vi "Mode 1 & 2.vi"() -> ()   [LabVIEW 2020]
uses:
  <vilib>/Platform/TimedLoop/XDataNode/timing_clust.ctl
  <vilib>/Platform/TimedLoop/XDataNode/nitl_modes.ctl
  <vilib>/Platform/TimedLoop/XDataNode/wakeup.ctl
  <vilib>/MakerHub/LINX/Public/Peripherals/Digital/Digital Read N Chans.vi
  <vilib>/MakerHub/LINX/Public/Peripherals/PWM/PWM Set Duty Cycle 1 Chan.vi
  <vilib>/MakerHub/LINX/Public/Peripherals/Digital/Digital Write N Chans.vi
  <vilib>/MakerHub/LINX/Private/Local IO/LinxDigitalRead.vi
  <vilib>/MakerHub/LINX/Public/Utilities/Check Channel.vi
  <vilib>/MakerHub/LINX/Private/Local IO/LinxDigitalWrite.vi
  <vilib>/MakerHub/LINX/Public/Utilities/Open Serial.vi
  <vilib>/MakerHub/LINX/Private/Utilties/Generate Error.vi
  <vilib>/MakerHub/LINX/Public/Peripherals/PWM/PWM Set Duty Cycle N Chans.vi
  <vilib>/MakerHub/LINX/Public/Sensors/Motion/Servo/Servo Open N Channels.vi
  <vilib>/MakerHub/LINX/Public/Sensors/Motion/Servo/Servo Set Pulse Width One Channel.vi
  <vilib>/MakerHub/LINX/Public/Sensors/Motion/Servo/Servo Close N Channels.vi
  <vilib>/platform/TimedLoop/XDataNode/XDataNode.xnode
  <vilib>/MakerHub/LINX/LMH-LINX.lvlib
  <vilib>/Platform/TimedLoop/XDataNode/XDNodeRunTimeDep.lvlib
  <vilib>/MakerHub/LINX/Public/Sensors/Motion/Servo/Servo.lvlib
panel:
  in  "Titik Stop":u16=110
  in  "Point":i32
  in  "Start Main Program":bool
  in  "Servo Magazine Pin":u8=3
  in  "Servo Slider 2 Pin":u8=4
  in  "Servo Slider 1 Pin":u8=5
  in  "Values":bool[](array[boolean])
  in  "Servo Slider 2 Angle":u16(knob)=82 scale=0.0..180.0
  in  "Servo Slider 1 Angle":u16(knob)=84 scale=0.0..180.0
  in  "Servo Magazine Angle":u16(knob)=110 scale=0.0..180.0
  in  "Slider Counter":dbl[](array[numeric])=[0.0, 0.0, 0.0, 13.0]
  out "Non-metal Workpiece":bool
  out "Metal Workpiece":bool
  out "Black Workpiece":bool
  out "White Workpiece":bool
  in  "Main Program":T1(array[cluster])=[{"Mode"=enum."Idle", "Limit"=enum."Tidak Ada", "Delay"=0, "Point"=0, "Row"=0}, {"Mode"=enum."Cek Ketersediaan", "Limit"=enum."Tidak Ada", "Delay"=500, "Point"=0, "Row"=1}, {"Mode"=enum."Workpiece Masuk", "Limit"=enum."Tidak Ada", "Delay"=0, "Point"=0, "Row"=2}, {"Mode"=enum."Cek Warna", "Limit"=enum."Tidak Ada", "Delay"=1000, "Point"=0, "Row"=3}, {"Mode"=enum."Cek Counter", "Limit"=enum."Tidak Ada", "Delay"=1000, "Point"=0, "Row"=4}, {"Mode"=enum."Servo Set", "Limit"=enum."Tidak Ada", "Delay"=1000, "Point"=0, "Row"=5}, {"Mode"=enum."Conveyor Jalan", "Limit"=enum."Tidak Ada", "Delay"=0, "Point"=0, "Row"=6}, {"Mode"=enum."Servo Reset", "Limit"=enum."Tidak Ada", "Delay"=1000, "Point"=0, "Row"=7}, {"Mode"=enum."Counter", "Limit"=enum."Tidak Ada", "Delay"=0, "Point"=0, "Row"=8}, {"Mode"=enum."Go To", "Limit"=enum."Tidak Ada", "Delay"=0, "Point"=1, "Row"=9}, {"Mode"=enum."Idle", "Limit"=enum."Tidak Ada", "Delay"=0, "Point"=0, "Row"=0}, {"Mode"=enum."Idle", "Limit"=enum."Tidak Ada", "Delay"=0, "Point"=0, "Row"=0}, {"Mode"=enum."Idle", "Limit"=enum."Tidak Ada", "Delay"=0, "Point"=0, "Row"=0}]
  in  "Stop Main Program":bool
  out "Row":i32
  in  "STOP":bool
  in  "Speed Pin":u8=2
  in  "Sensor Pin":u8[](array[numeric])=[30, 32, 50, 34, 36, 38]
  out "Sensor Value":bool[](array[boolean])
  in  "Duty Cycle":dbl(knob) scale=0.0..100.0
  out "Device Name":string
  in  "Arduino Port":refnum<visa-resource-name>="N/A"
  # "LOW COST MPS SORTING BASED ARDUINO"
  # "MAIN PROGRAM"
  # "PROJECT MONITOR"
  # "MODE 1"
  # "Index Array Counter\n\n-----Mode 1-----\n0. White Workpiece          \n1. Black Workpiece\n\n-----Mode 2-----\n0. Metal Workpiece\n1. Non-metal Workpiece"
  # "MODE 2"
  # "INPUT/OUTPUT CONTROL"
  # "Index Array Input Sensor\n\n0. IR Sensor Stack Magazine\n1. IR Sensor B/W Check\n2. Inductive Proximity Sensor\n3. IR Sensor Slider 1\n4. IR Sensor Slider 2\n5. IR Sensor Slider 3"
  # "Mechatronics Engineering 2nd Generation - Vocational High School 2 Bojonegoro"
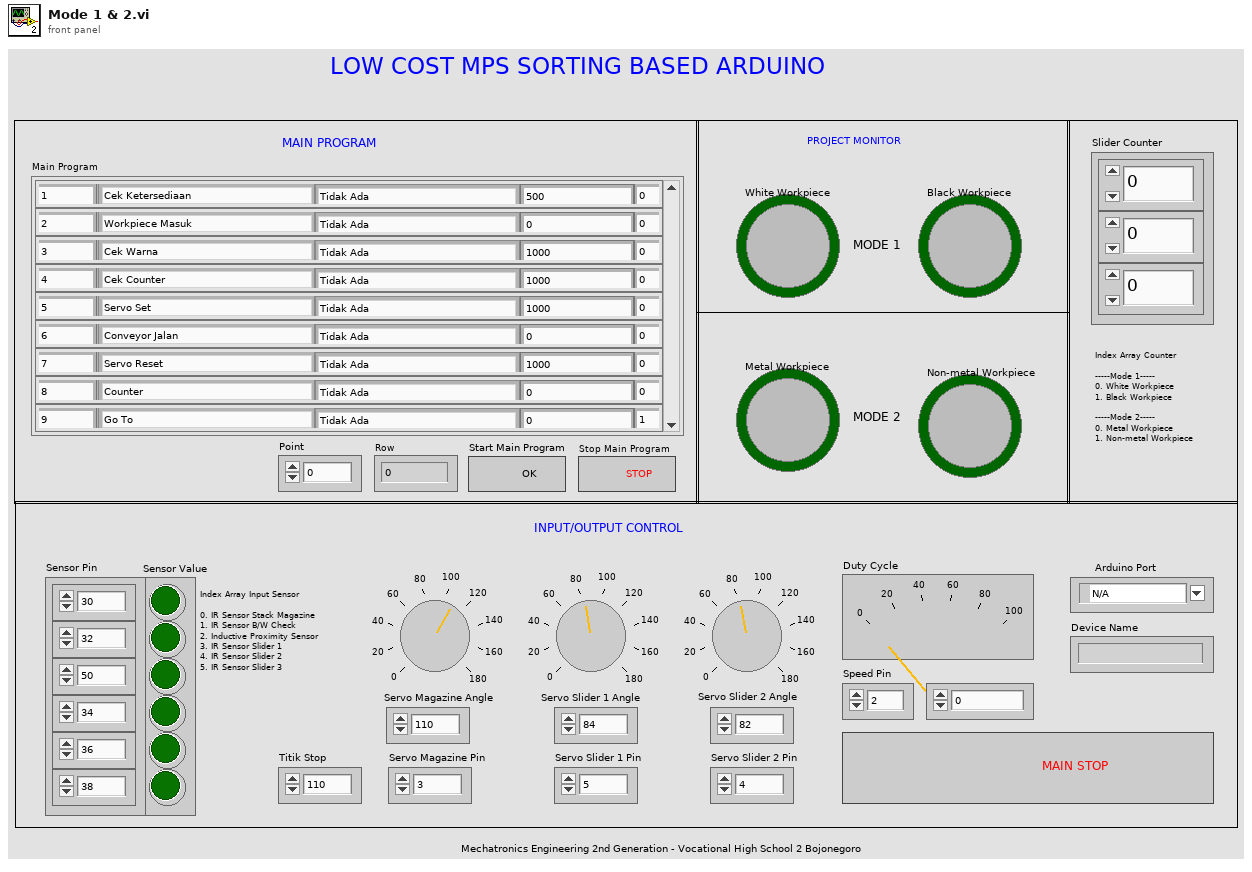
[diagram p1: front panel]
types:
  T1 = cluster{"Mode":enum16{"Idle", "Cek Ketersediaan", "Workpiece Masuk", "Cek Bahan", "Cek Warna", "Servo Set", "Conveyor Jalan", "Servo Reset", "Counter", "Cek Counter", "Go To"}, "Limit":enum16{"Tidak Ada", "Sensor Slider"}, "Delay":i32, "Point":i32, "Row":i32}[]
  T2 = typedef "XDNodeRunTimeDep.lvlib/timing_clust.ctl" = cluster{"Expected End [f-1]":u64, "Actual End [f-1]":u64, "Finished Late? [f-1]":bool, "Expected End [i-1]":u64, "Actual End [i-1]":u64, "Finished Late? [i-1]":bool, "Expected Start [i]":u64, "Actual Start [i]":u64, "Expected Start [f]":u64, "Actual Start [f]":u64, "Source Name":string, "Structure Name":string, "Period":i64, "Deadline":i64, "Offset":i64, "Start":i64, "Priority":i32, "Timeout":i32, "Mode":T3, "Wakeup Reason":T4, "Error":errorcluster, "Source Type":string, "Secondary Source Type":string, "Global End Time":u64, "Global Start Time":u64, "Frame Duration":u64, "Iteration Duration":u64, "Assigned CPU":i32, "I/O Scan Engine Mode":u32}
  T3 = typedef "XDNodeRunTimeDep.lvlib/nitl_modes.ctl" = enum32{"No Change", "Process missed periods, maintain original phase", "Discard missed periods, maintain original phase", "Process missed periods, ignore original phase", "Discard missed periods, ignore original phase"}
  T4 = typedef "XDNodeRunTimeDep.lvlib/wakeup.ctl" = enum32{"Normal", "Aborted", "Asynchronous wakeup", "Timing source error", "Timed loop error", "Timeout"}
  T5 = cluster{"Mode":enum16{"Idle", "Cek Ketersediaan", "Workpiece Masuk", "Cek Bahan", "Cek Warna", "Servo Set", "Conveyor Jalan", "Servo Reset", "Counter", "Cek Counter", "Go To"}, "Limit":enum16{"Tidak Ada", "Sensor Slider"}, "Delay":i32, "Point":i32, "Row":i32}
  T6 = enum16{"Idle", "Cek Ketersediaan", "Workpiece Masuk", "Cek Bahan", "Cek Warna", "Servo Set", "Conveyor Jalan", "Servo Reset", "Counter", "Cek Counter", "Go To"}
  T7 = typedef "LMH-LINX.lvlib/LINX Ref.ctl" = cluster{"IO":T8, "Interface":T9, "LINX Device Config":T10}
  T8 = typedef "LMH-LINX.lvlib/Platform.ctl" = enum16{"Remote", "Local"}
  T9 = typedef "LMH-LINX.lvlib/Interface.ctl" = enum16{"Serial", "TCP"}
  T10 = typedef "LMH-LINX.lvlib/Device.lvlib/LINX Device Config.ctl" = cluster{"Interface":T9, "COM Port":refnum<visa-resource-name>, "TCP Configuration":T11, "Device Family":u8, "Device ID":u8, "Device Name":string, "TCP Ref":refnum<k5>, "Channels":T12}
  T11 = typedef "LMH-LINX.lvlib/Device.lvlib/TCP Config.ctl" = cluster{"IP Address":string, "Port":u16}
  T12 = typedef "LMH-LINX.lvlib/Channels.ctl" = cluster{"DI":u8[], "DO":u8[], "AI":u8[], "AO":u8[], "PWM":u8[], "QE":u8[], "UART":u8[], "I2C 2":u8[], "SPI":u8[], "CAN":u8[], "Servo":u8[], "AI Ref (V)":dbl, "AI Resolution (Bits)":u8, "AO Ref (V)":dbl, "AO Resolution (Bits)":u8}
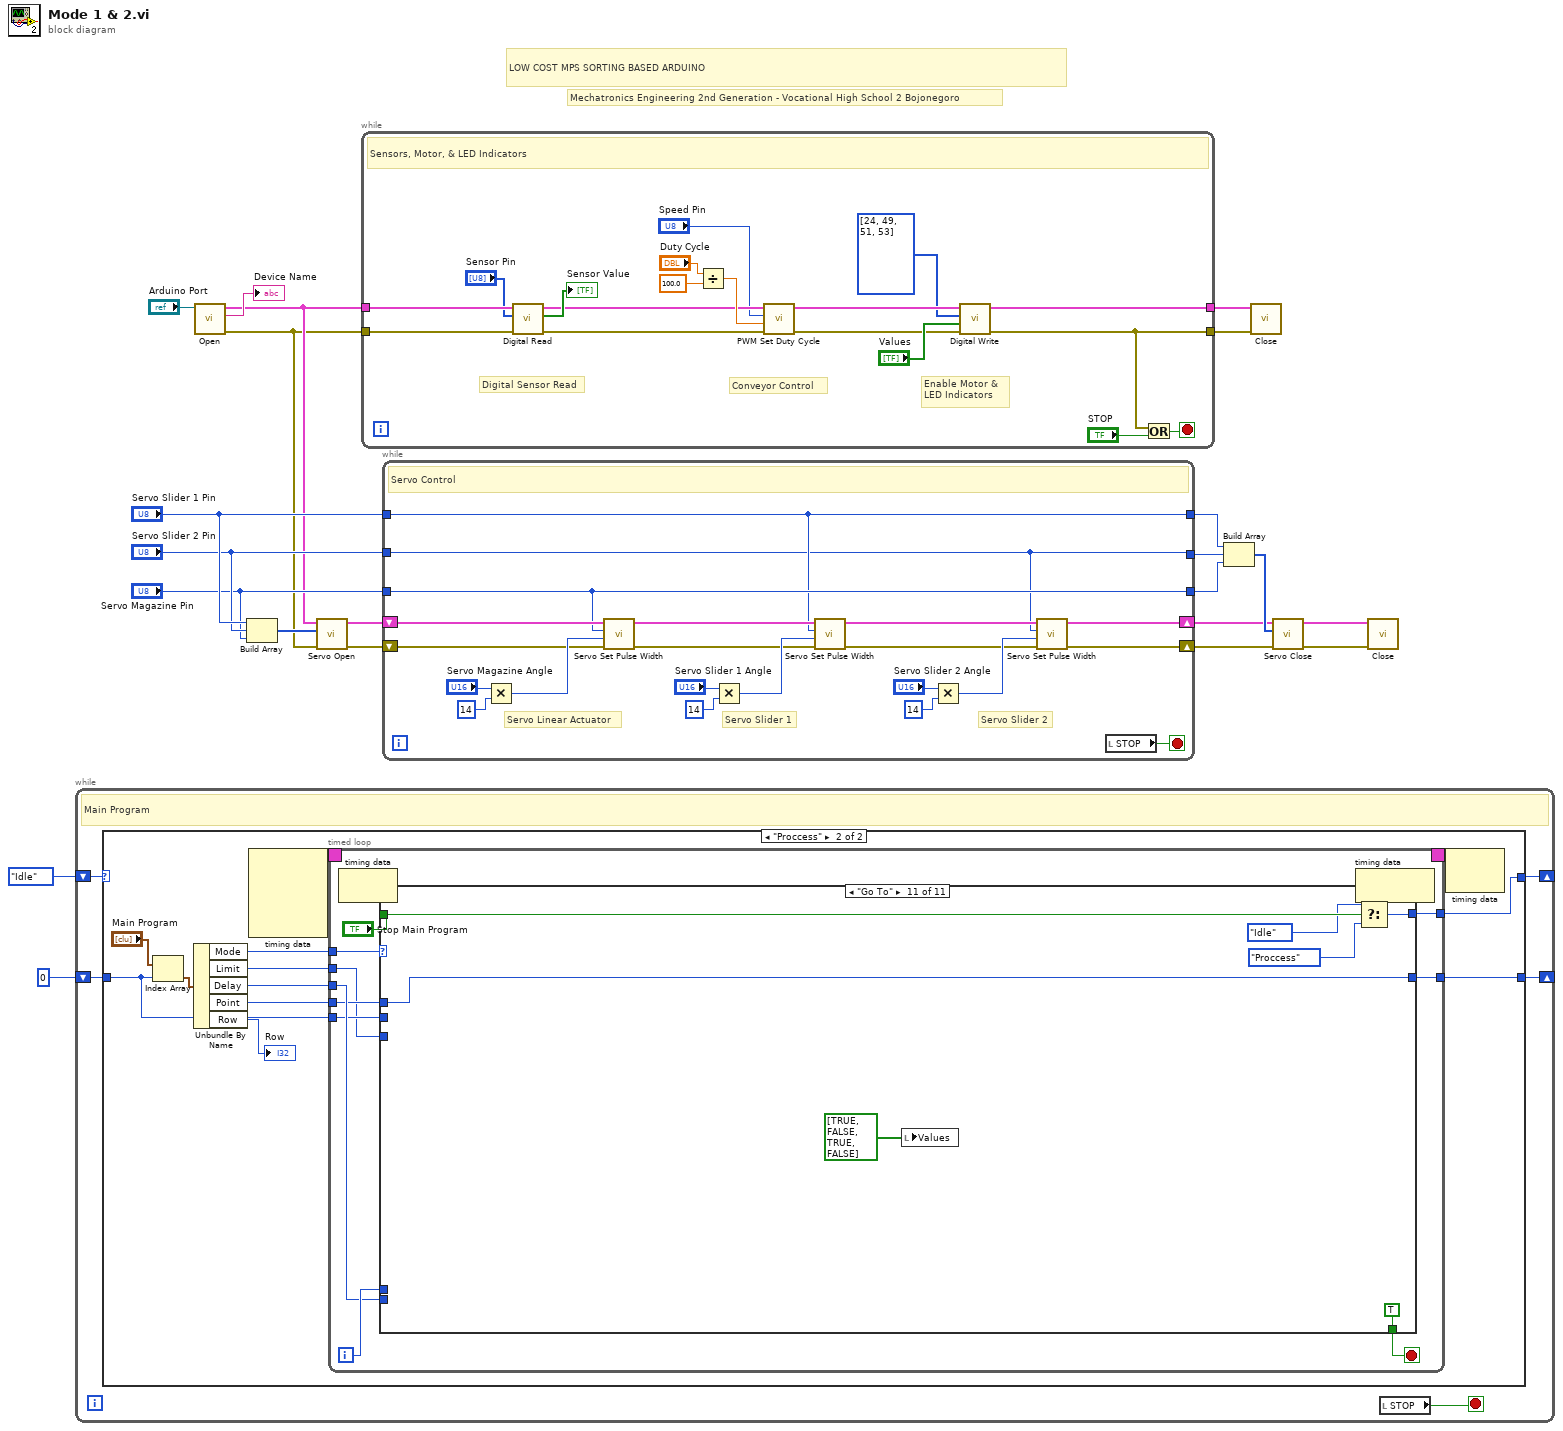
[diagram p0: block diagram]
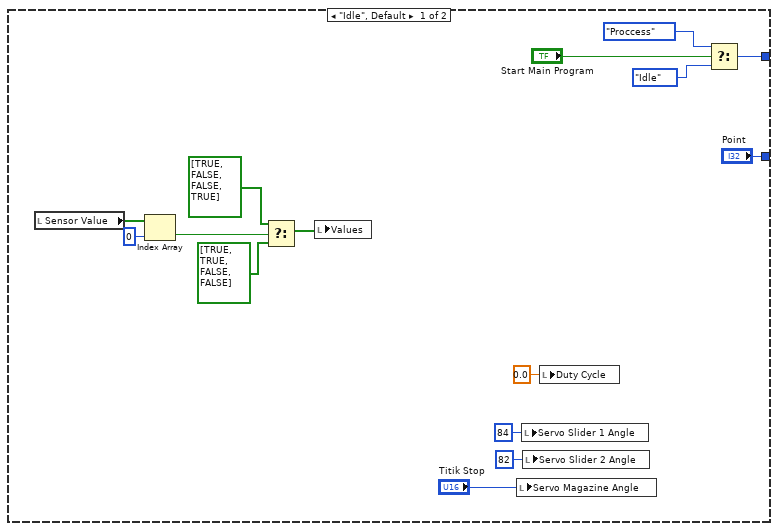
[diagram p2: hidden frame]
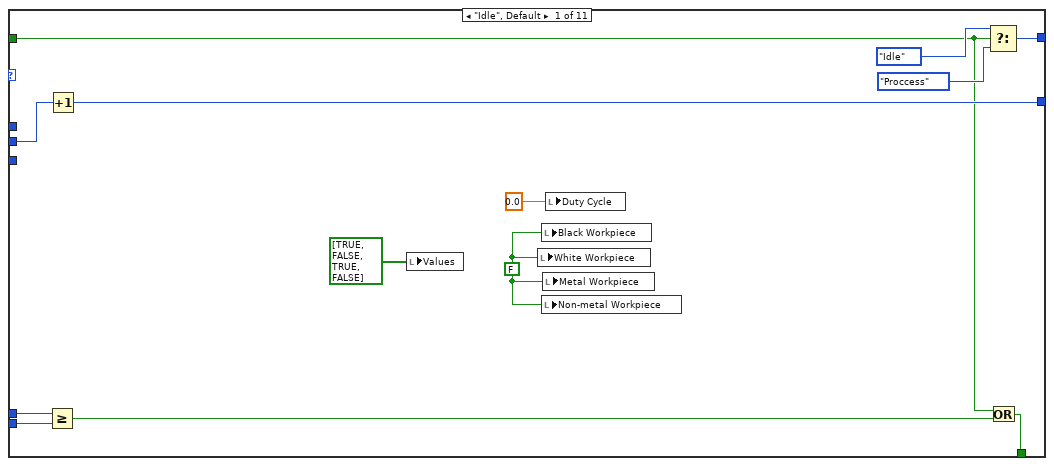
[diagram p3: hidden frame]
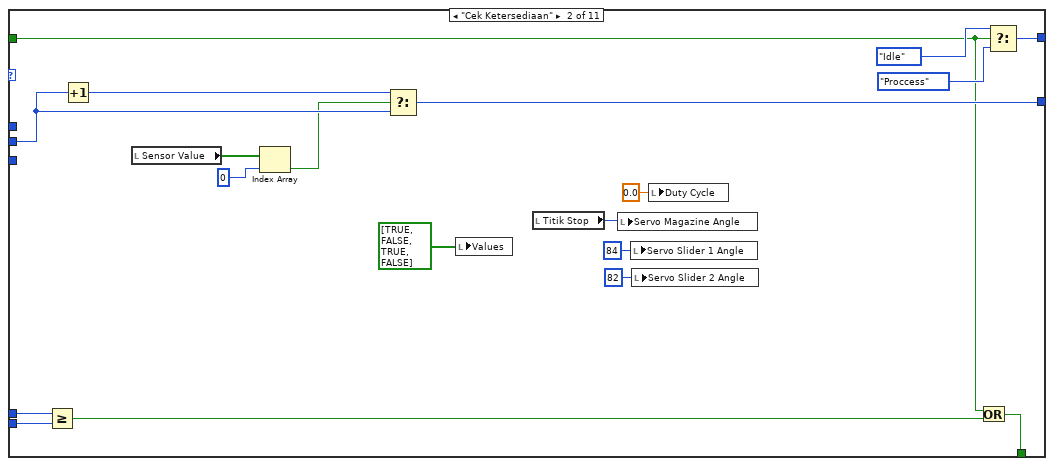
[diagram p4: hidden frame]
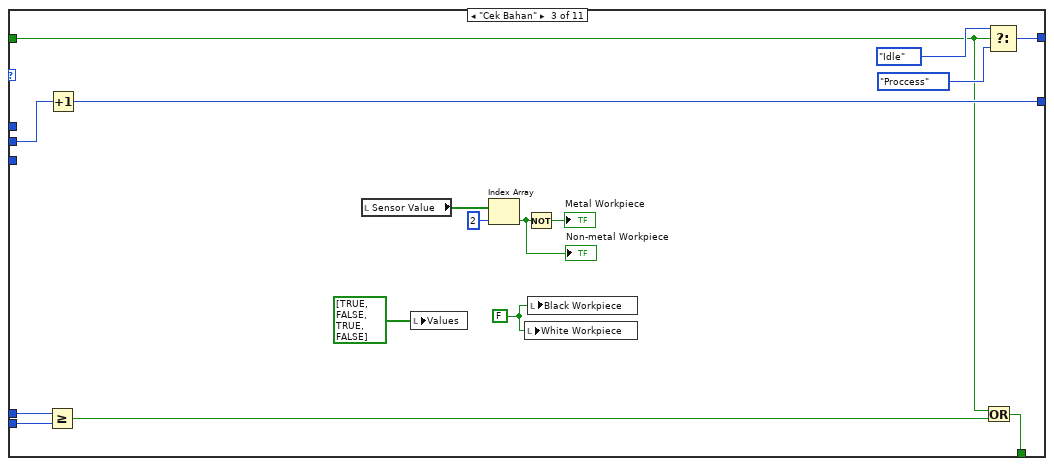
[diagram p5: hidden frame]
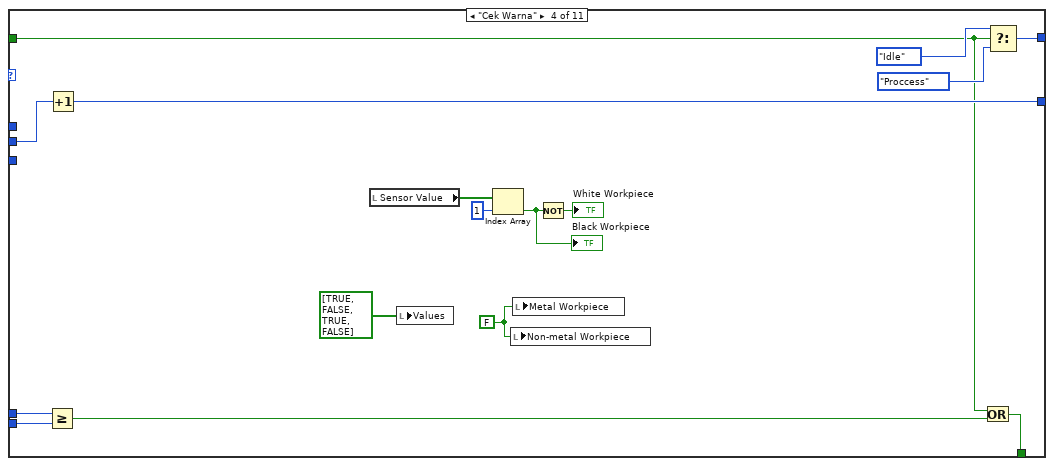
[diagram p6: hidden frame]
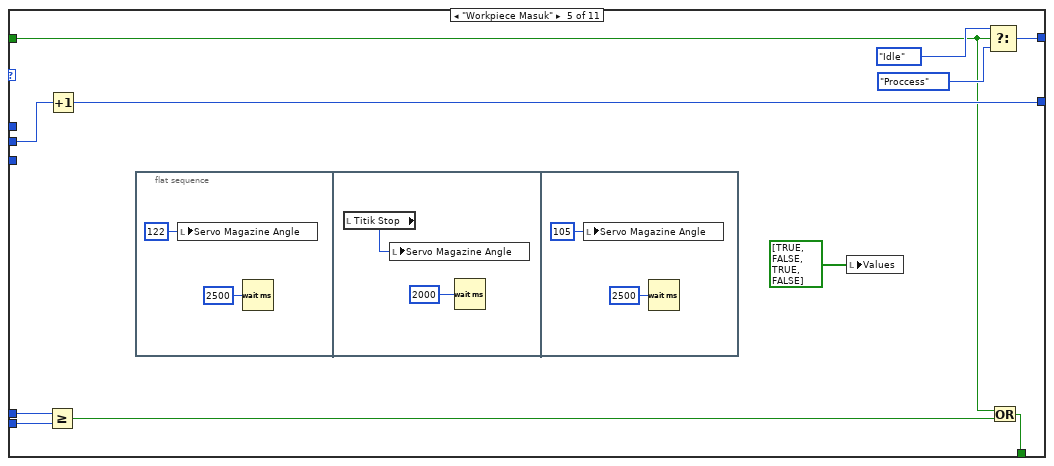
[diagram p7: hidden frame]
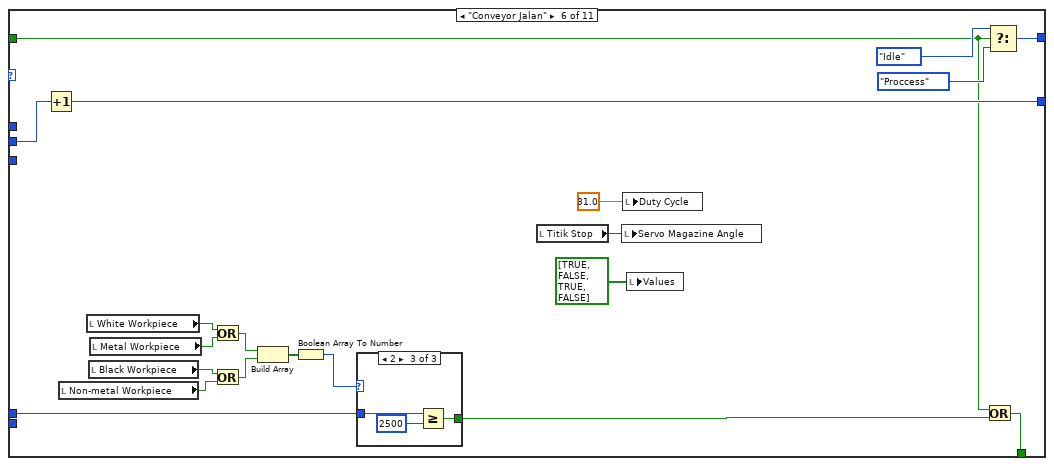
[diagram p8: hidden frame]
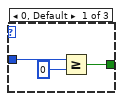
[diagram p9: hidden frame]
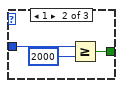
[diagram p10: hidden frame]
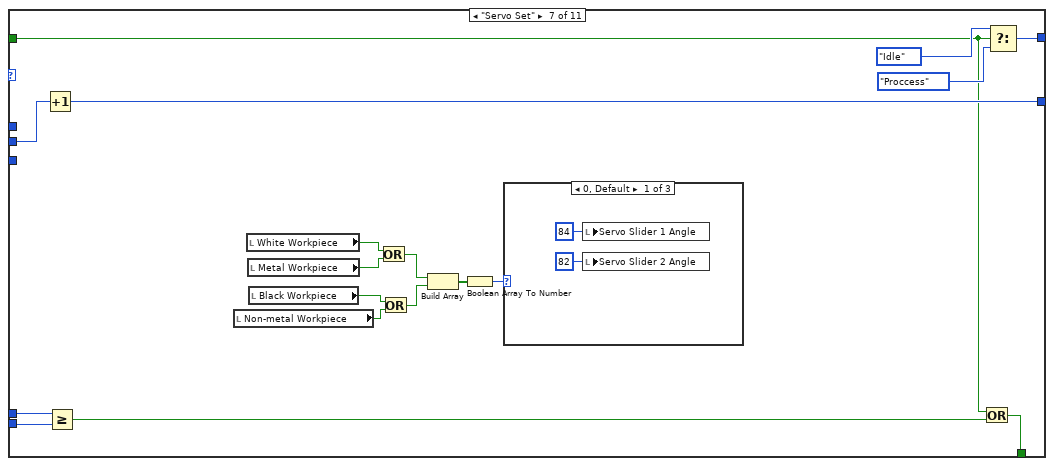
[diagram p11: hidden frame]
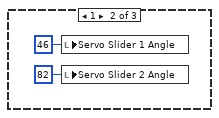
[diagram p12: hidden frame]
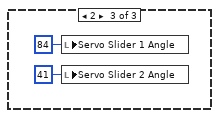
[diagram p13: hidden frame]
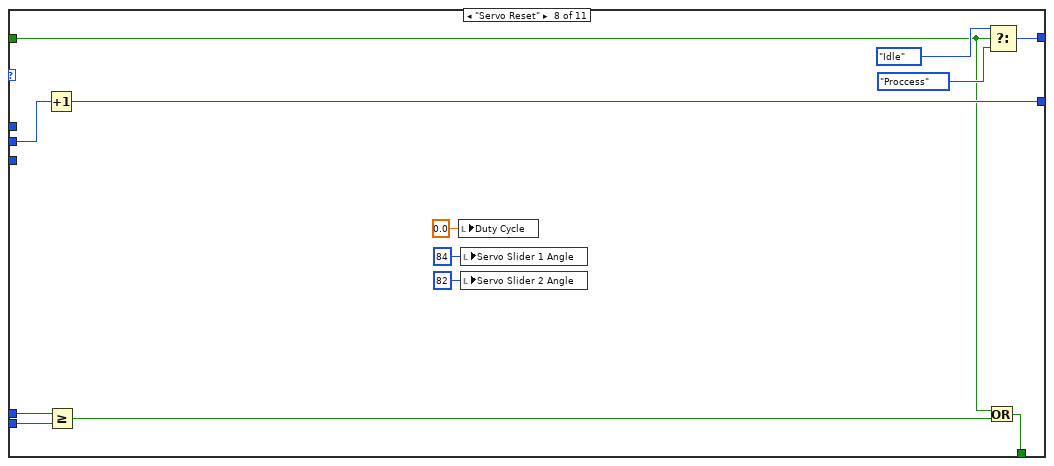
[diagram p14: hidden frame]
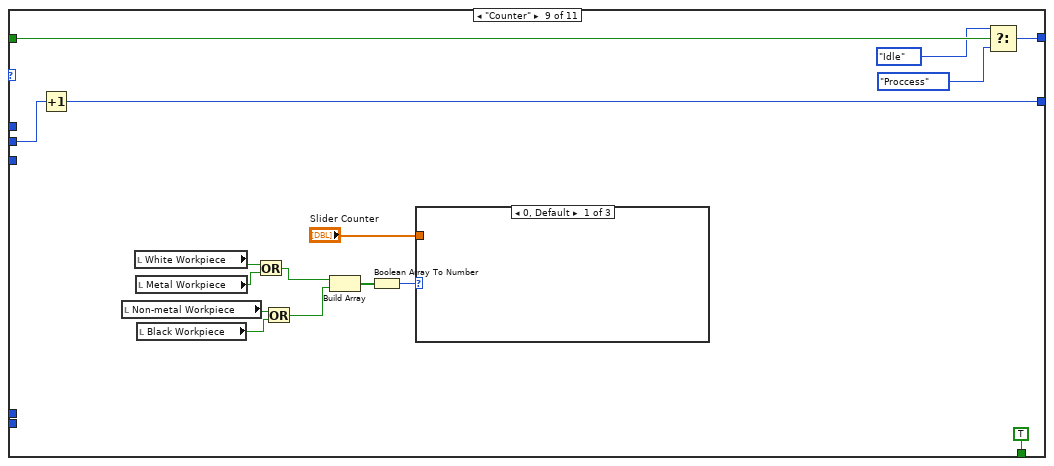
[diagram p15: hidden frame]
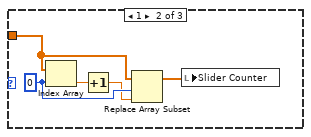
[diagram p16: hidden frame]
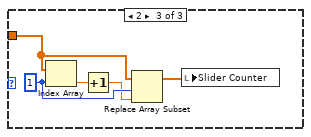
[diagram p17: hidden frame]
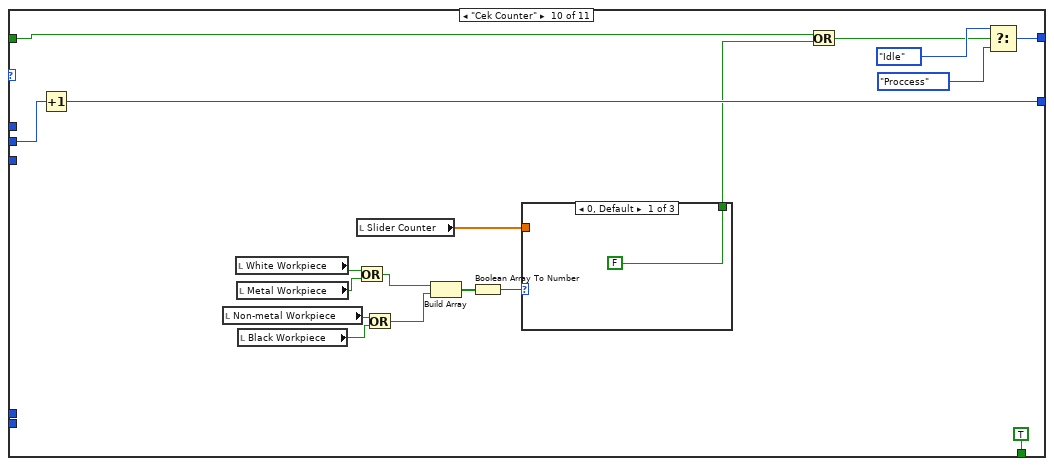
[diagram p18: hidden frame]
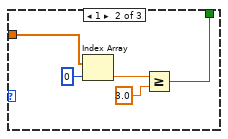
[diagram p19: hidden frame]
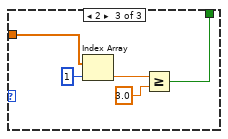
[diagram p20: hidden frame]
diagram:
  # "Mechatronics Engineering 2nd Generation - Vocational High School 2 Bojonegoro"
  # "LOW COST MPS SORTING BASED ARDUINO"
  n1 = while {
    shift-right: [w26] -> _
    shift-left: enum16{"Idle", "Proccess"}."Idle" -> [w23]
    shift-right: [w24] -> _
    shift-left: 0 ("index") -> [w25]
    stop <- w27 stop-if-true
    # "Main Program"
    n2 = case shown="\"Proccess\"" w23 {
      tunnel: [w42 w51] -> w26
      tunnel: w25 -> [_ w50]
      tunnel: ["Point" w49] -> w24
      frame "Idle", Default {
        n3 = local read "Sensor Value"() -> (w34:bool[])
        n4 = Index Array(array=w34, index=0) -> (element=w32:bool)
        n5 = Select(t=bool[] [TRUE, FALSE, FALSE, TRUE] ("Values"), s=w32, f=bool[] [TRUE, TRUE, FALSE, FALSE]) -> (s? t:f=w31:bool[])
        n6 = local write "Values"(w31) -> ()
        n7 = local write "Servo Magazine Angle"("Titik Stop") -> ()
        n8 = local write "Servo Slider 1 Angle"(u16 84 ("Servo Slider 1 Angle")) -> ()
        n9 = local write "Servo Slider 2 Angle"(u16 82 ("Servo Slider 2 Angle")) -> ()
        n10 = local write "Duty Cycle"(0.0 ("Duty Cycle")) -> ()
        n11 = Select(t=enum16{"Idle", "Proccess"}."Proccess", s="Start Main Program", f=enum16{"Idle", "Proccess"}."Idle") -> (s? t:f=w42:enum16{"Idle", "Proccess"})
      }
      frame "Proccess" {
        n12 = Index Array(array="Main Program", index=w50) -> (element=w54:T5)
        n13 = Unbundle By Name(w54) -> ("Mode"=w53:T6, "Limit"=w45:enum16{"Tidak Ada", "Sensor Slider"}, "Delay"=w52:i32, "Point"=w46:i32, "Row"=→"Row":i32)
        n14 = node-c288() -> (w48:T2)  [unwired: 4 in]
        n15 = timed-loop {
          tunnel: w53 -> [w64]
          tunnel: w52 -> [w62]
          tunnel: [w60] -> w51
          tunnel: w50 -> [w59]
          tunnel: [w58] -> w49
          timing: w48 -> [_]
          timing-out: [_] -> w47
          tunnel: w46 -> [w57]
          tunnel: w45 -> [w56]
          i -> [w63]
          stop <- w61 stop-if-true
          n16 = node-c288() -> ()  [unwired: 1 in, 1 out]
          n17 = case shown="\"Go To\"" w64 {
            tunnel: w63 -> [w73 w94 w110 w126 w135 w152 w189 w208 _ _ _]
            tunnel: w62 -> [w74 w95 w111 w127 w136 _ w188 w207 _ _ _]
            tunnel: [w69 w88 w102 w118 w134 w162 w179 w203 TRUE TRUE TRUE] -> w61
            tunnel: "Stop Main Program" -> [w67 w86 w100 w116 w132 w161 w178 w201 w228 w241 w274]
            tunnel: [w79 w98 w114 w130 w141 w167 w194 w213 w229 w257 w275] -> w60
            tunnel: w59 -> [w76 w89 w107 w123 w138 w163 w191 w210 w225 w254 _]
            tunnel: [w75 w91 w106 w122 w137 w164 w190 w209 w224 w253 w271] -> w58
            tunnel: w57 -> [_ _ _ _ _ _ _ _ _ _ w271]
            tunnel: w56 -> [_ _ _ _ _ _ _ _ _ _ _]
            frame "Idle", Default {
              w72 = FALSE
              n18 = Greater Or Equal?(x=w73, y=w74) -> (x >= y?=w68:bool)
              n19 = Increment(x=w76) -> (x+1=w75:i32)
              n20 = local write "Values"(bool[] [TRUE, FALSE, TRUE, FALSE] ("Values")) -> ()
              n21 = local write "White Workpiece"(w72) -> ()
              n22 = local write "Black Workpiece"(w72) -> ()
              n23 = local write "Non-metal Workpiece"(w72) -> ()
              n24 = local write "Metal Workpiece"(w72) -> ()
              n25 = local write "Duty Cycle"(0.0 ("Duty Cycle (0-1)")) -> ()
              n26 = Select(t=enum16{"Idle", "Proccess"}."Idle", s=w67, f=enum16{"Idle", "Proccess"}."Proccess") -> (s? t:f=w79:enum16{"Idle", "Proccess"})
              n27 = Or(x=w67, y=w68) -> (x .or. y?=w69:bool)
            }
            frame "Cek Ketersediaan" {
              n28 = Greater Or Equal?(x=w94, y=w95) -> (x >= y?=w87:bool)
              n29 = Increment(x=w89) -> (x+1=w90:i32)
              n30 = local read "Sensor Value"() -> (w93:bool[])
              n31 = Index Array(array=w93, index=0) -> (element=w85:bool)
              n32 = Select(t=w90, s=w85, f=w89) -> (s? t:f=w91:i32)
              n33 = local write "Values"(bool[] [TRUE, FALSE, TRUE, FALSE] ("Values")) -> ()
              n34 = local read "Titik Stop"() -> (w80:u16)
              n35 = local write "Servo Magazine Angle"(w80) -> ()
              n36 = local write "Servo Slider 1 Angle"(u16 84 ("Servo Slider 1 Angle")) -> ()
              n37 = local write "Servo Slider 2 Angle"(u16 82 ("Servo Slider 2 Angle")) -> ()
              n38 = local write "Duty Cycle"(0.0 ("Duty Cycle")) -> ()
              n39 = Or(x=w86, y=w87) -> (x .or. y?=w88:bool)
              n40 = Select(t=enum16{"Idle", "Proccess"}."Idle", s=w86, f=enum16{"Idle", "Proccess"}."Proccess") -> (s? t:f=w98:enum16{"Idle", "Proccess"})
            }
            frame "Cek Bahan" {
              w105 = FALSE
              n41 = Greater Or Equal?(x=w110, y=w111) -> (x >= y?=w101:bool)
              n42 = Increment(x=w107) -> (x+1=w106:i32)
              n43 = local read "Sensor Value"() -> (w109:bool[])
              n44 = local write "Values"(bool[] [TRUE, FALSE, TRUE, FALSE] ("Values")) -> ()
              n45 = Index Array(array=w109, index=2) -> (element=w103:bool)
              "Non-metal Workpiece" <- w103
              n46 = local write "White Workpiece"(w105) -> ()
              n47 = Not(x=w103) -> (.not. x?=→"Metal Workpiece":bool)
              n48 = local write "Black Workpiece"(w105) -> ()
              n49 = Or(x=w100, y=w101) -> (x .or. y?=w102:bool)
              n50 = Select(t=enum16{"Idle", "Proccess"}."Idle", s=w100, f=enum16{"Idle", "Proccess"}."Proccess") -> (s? t:f=w114:enum16{"Idle", "Proccess"})
            }
            frame "Cek Warna" {
              w121 = FALSE
              n51 = Greater Or Equal?(x=w126, y=w127) -> (x >= y?=w117:bool)
              n52 = Increment(x=w123) -> (x+1=w122:i32)
              n53 = local read "Sensor Value"() -> (w125:bool[])
              n54 = local write "Values"(bool[] [TRUE, FALSE, TRUE, FALSE] ("Values")) -> ()
              n55 = Index Array(array=w125, index=1) -> (element=w119:bool)
              "Black Workpiece" <- w119
              n56 = local write "Non-metal Workpiece"(w121) -> ()
              n57 = local write "Metal Workpiece"(w121) -> ()
              n58 = Not(x=w119) -> (.not. x?=→"White Workpiece":bool)
              n59 = Or(x=w116, y=w117) -> (x .or. y?=w118:bool)
              n60 = Select(t=enum16{"Idle", "Proccess"}."Idle", s=w116, f=enum16{"Idle", "Proccess"}."Proccess") -> (s? t:f=w130:enum16{"Idle", "Proccess"})
            }
            frame "Workpiece Masuk" {
              n61 = Greater Or Equal?(x=w135, y=w136) -> (x >= y?=w133:bool)
              n62 = Increment(x=w138) -> (x+1=w137:i32)
              n63 = flat-sequence {
                frame #0 {
                  n64 = local write "Servo Magazine Angle"(u16 122 ("Servo Magazine Angle")) -> ()
                  n65 = Wait (ms)(milliseconds to wait=u32 2500) -> ()  [unwired: 1 out]
                }
                frame #1 {
                  n66 = local read "Titik Stop"() -> (w144:u16)
                  n67 = local write "Servo Magazine Angle"(w144) -> ()
                  n68 = Wait (ms)(milliseconds to wait=u32 2000) -> ()  [unwired: 1 out]
                }
                frame #2 {
                  n69 = local write "Servo Magazine Angle"(u16 105 ("Servo Magazine Angle")) -> ()
                  n70 = Wait (ms)(milliseconds to wait=u32 2500) -> ()  [unwired: 1 out]
                }
              }
              n71 = local write "Values"(bool[] [TRUE, FALSE, TRUE, FALSE] ("Values")) -> ()
              n72 = Select(t=enum16{"Idle", "Proccess"}."Idle", s=w132, f=enum16{"Idle", "Proccess"}."Proccess") -> (s? t:f=w141:enum16{"Idle", "Proccess"})
              n73 = Or(x=w132, y=w133) -> (x .or. y?=w134:bool)
            }
            frame "Conveyor Jalan" {
              n74 = Increment(x=w163) -> (x+1=w164:i32)
              n75 = local read "Non-metal Workpiece"() -> (w157:bool)
              n76 = local read "White Workpiece"() -> (w159:bool)
              n77 = local read "Black Workpiece"() -> (w158:bool)
              n78 = local read "Metal Workpiece"() -> (w160:bool)
              n79 = Or(x=w159, y=w160) -> (x .or. y?=w156:bool)
              n80 = Or(x=w158, y=w157) -> (x .or. y?=w155:bool)
              n81 = Build Array(w156, w155) -> (w154:bool[])
              n82 = Boolean Array To Number(Boolean array=w154) -> (number=w153:u32)
              n83 = case shown="2" w153 {
                tunnel: w152 -> [w170 w173 w176]
                tunnel: [w169 w172 w175] -> w151
                frame 0, Default {
                  n84 = Greater Or Equal?(x=w170, y=0) -> (x >= y?=w169:bool)
                }
                frame 1 {
                  n85 = Greater Or Equal?(x=w173, y=2000) -> (x >= y?=w172:bool)
                }
                frame 2 {
                  n86 = Greater Or Equal?(x=w176, y=2500) -> (x >= y?=w175:bool)
                }
              }
              n87 = local read "Titik Stop"() -> (w148:u16)
              n88 = local write "Servo Magazine Angle"(w148) -> ()
              n89 = local write "Duty Cycle"(31.0 ("Duty Cycle (0-1)")) -> ()
              n90 = local write "Values"(bool[] [TRUE, FALSE, TRUE, FALSE] ("Values")) -> ()
              n91 = Or(x=w161, y=w151) -> (x .or. y?=w162:bool)
              n92 = Select(t=enum16{"Idle", "Proccess"}."Idle", s=w161, f=enum16{"Idle", "Proccess"}."Proccess") -> (s? t:f=w167:enum16{"Idle", "Proccess"})
            }
            frame "Servo Set" {
              n93 = Increment(x=w191) -> (x+1=w190:i32)
              n94 = Greater Or Equal?(x=w189, y=w188) -> (x >= y?=w177:bool)
              n95 = local read "Non-metal Workpiece"() -> (w184:bool)
              n96 = local read "White Workpiece"() -> (w187:bool)
              n97 = local read "Metal Workpiece"() -> (w186:bool)
              n98 = local read "Black Workpiece"() -> (w185:bool)
              n99 = Or(x=w187, y=w186) -> (x .or. y?=w183:bool)
              n100 = Or(x=w185, y=w184) -> (x .or. y?=w182:bool)
              n101 = Build Array(w183, w182) -> (w181:bool[])
              n102 = Boolean Array To Number(Boolean array=w181) -> (number=w180:u32)
              n103 = case shown="0, Default" w180 {
                frame 0, Default {
                  n104 = local write "Servo Slider 1 Angle"(u16 84 ("Servo Slider 1 Angle")) -> ()
                  n105 = local write "Servo Slider 2 Angle"(u16 82 ("Servo Slider 2 Angle")) -> ()
                }
                frame 1 {
                  n106 = local write "Servo Slider 1 Angle"(u16 46 ("Servo Slider 1 Angle")) -> ()
                  n107 = local write "Servo Slider 2 Angle"(u16 82 ("Servo Slider 2 Angle")) -> ()
                }
                frame 2 {
                  n108 = local write "Servo Slider 1 Angle"(u16 84 ("Servo Slider 1 Angle")) -> ()
                  n109 = local write "Servo Slider 2 Angle"(u16 41 ("Servo Slider 2 Angle")) -> ()
                }
              }
              n110 = Or(x=w178, y=w177) -> (x .or. y?=w179:bool)
              n111 = Select(t=enum16{"Idle", "Proccess"}."Idle", s=w178, f=enum16{"Idle", "Proccess"}."Proccess") -> (s? t:f=w194:enum16{"Idle", "Proccess"})
            }
            frame "Servo Reset" {
              n112 = Increment(x=w210) -> (x+1=w209:i32)
              n113 = Greater Or Equal?(x=w208, y=w207) -> (x >= y?=w202:bool)
              n114 = local write "Duty Cycle"(0.0 ("Duty Cycle")) -> ()
              n115 = local write "Servo Slider 1 Angle"(u16 84 ("Servo Slider 1 Angle")) -> ()
              n116 = local write "Servo Slider 2 Angle"(u16 82 ("Servo Slider 2 Angle")) -> ()
              n117 = Or(x=w201, y=w202) -> (x .or. y?=w203:bool)
              n118 = Select(t=enum16{"Idle", "Proccess"}."Idle", s=w201, f=enum16{"Idle", "Proccess"}."Proccess") -> (s? t:f=w213:enum16{"Idle", "Proccess"})
            }
            frame "Counter" {
              n119 = Increment(x=w225) -> (x+1=w224:i32)
              n120 = local read "Non-metal Workpiece"() -> (w217:bool)
              n121 = local read "White Workpiece"() -> (w219:bool)
              n122 = local read "Metal Workpiece"() -> (w218:bool)
              n123 = local read "Black Workpiece"() -> (w216:bool)
              n124 = Or(x=w219, y=w218) -> (x .or. y?=w215:bool)
              n125 = Or(x=w217, y=w216) -> (x .or. y?=w214:bool)
              n126 = Build Array(w215, w214) -> (w222:bool[])
              n127 = Boolean Array To Number(Boolean array=w222) -> (number=w221:u32)
              n128 = case shown="0, Default" w221 {
                tunnel: "Slider Counter" -> [_ w230 w235]
                frame 0, Default {
                }
                frame 1 {
                  w232 = 0 ("index")
                  n129 = Index Array(array=w230, index=w232) -> (element=w234:dbl)
                  n130 = Increment(x=w234) -> (x+1=w231:dbl)
                  n131 = Replace Array Subset(array=w230, new element=w231, index=w232) -> (w233:dbl[])
                  n132 = local write "Slider Counter"(w233) -> ()
                }
                frame 2 {
                  w237 = 1 ("index")
                  n133 = Index Array(array=w235, index=w237) -> (element=w239:dbl)
                  n134 = Increment(x=w239) -> (x+1=w236:dbl)
                  n135 = Replace Array Subset(array=w235, new element=w236, index=w237) -> (w238:dbl[])
                  n136 = local write "Slider Counter"(w238) -> ()
                }
              }
              n137 = Select(t=enum16{"Idle", "Proccess"}."Idle", s=w228, f=enum16{"Idle", "Proccess"}."Proccess") -> (s? t:f=w229:enum16{"Idle", "Proccess"})
            }
            frame "Cek Counter" {
              n138 = Increment(x=w254) -> (x+1=w253:i32)
              n139 = local read "Non-metal Workpiece"() -> (w247:bool)
              n140 = local read "White Workpiece"() -> (w249:bool)
              n141 = local read "Metal Workpiece"() -> (w248:bool)
              n142 = local read "Black Workpiece"() -> (w246:bool)
              n143 = local read "Slider Counter"() -> (w243:dbl[])
              n144 = Or(x=w249, y=w248) -> (x .or. y?=w245:bool)
              n145 = Or(x=w247, y=w246) -> (x .or. y?=w244:bool)
              n146 = Build Array(w245, w244) -> (w251:bool[])
              n147 = Boolean Array To Number(Boolean array=w251) -> (number=w250:u32)
              n148 = case shown="0, Default" w250 {
                tunnel: w243 -> [_ w262 w267]
                tunnel: [FALSE w259 w264] -> w240
                frame 0, Default {
                }
                frame 1 {
                  n149 = Index Array(array=w262, index=0) -> (element=w261:dbl)
                  n150 = Greater Or Equal?(x=w261, y=3.0) -> (x >= y?=w259:bool)
                }
                frame 2 {
                  n151 = Index Array(array=w267, index=1) -> (element=w266:dbl)
                  n152 = Greater Or Equal?(x=w266, y=3.0) -> (x >= y?=w264:bool)
                }
              }
              n153 = Or(x=w241, y=w240) -> (x .or. y?=w242:bool)
              n154 = Select(t=enum16{"Idle", "Proccess"}."Idle", s=w242, f=enum16{"Idle", "Proccess"}."Proccess") -> (s? t:f=w257:enum16{"Idle", "Proccess"})
            }
            frame "Go To" {
              n155 = local write "Values"(bool[] [TRUE, FALSE, TRUE, FALSE] ("Values")) -> ()
              n156 = Select(t=enum16{"Idle", "Proccess"}."Idle", s=w274, f=enum16{"Idle", "Proccess"}."Proccess") -> (s? t:f=w275:enum16{"Idle", "Proccess"})
            }
          }
          n157 = node-c288() -> ()  [unwired: 1 in, 1 out]
        }
        n158 = node-c288(w47) -> ()  [unwired: 1 out]
      }
    }
    n159 = local read "STOP"() -> (w27:bool)
  }
  n160 = call-poly <vilib>:"Open.vi"("Serial Port"="Arduino Port") -> ("Error Out"=w1:errorcluster, "Device Name"=→"Device Name":string, "LINX Resource"=w2:T7)  [unwired: 8 in]
  n161 = Build Array("Servo Slider 1 Pin", "Servo Slider 2 Pin", "Servo Magazine Pin") -> (w13:u8[])
  n162 = call-poly <vilib>:"Servo Open.vi"("Error In"=w1, "Servo Channels"=w13, "LINX Resource"=w2) -> ("Error Out"=w11:errorcluster, "LINX Resource"=w12:T7)  [unwired: 7 in]
  n163 = while {
    tunnel: w2 -> [w293]
    tunnel: [w283] -> w22
    tunnel: [w284] -> w21
    tunnel: w1 -> [w292]
    stop <- w295 stop-if-true
    # "Enable Motor &\nLED Indicators"
    # "Conveyor Control"
    # "Digital Sensor Read"
    # "Sensors, Motor, & LED Indicators"
    n164 = call-poly <vilib>:"Digital Read.vi"("Error In"=w292, "DI Channels"="Sensor Pin", "LINX Resource"=w293) -> ("Error Out"=w281:errorcluster, "Values"=→"Sensor Value":bool[], "LINX Resource"=w282:T7)  [unwired: 6 in]
    n165 = Divide(x="Duty Cycle", y=100.0) -> (x/y=w289:dbl)
    n166 = call-poly <vilib>:"PWM Set Duty Cycle.vi"("Error In"=w281, "Duty Cycle (0-1)"=w289, "PWM Channel"="Speed Pin", "LINX Resource"=w282) -> ("Error Out"=w285:errorcluster, "LINX Resource"=w286:T7)  [unwired: 6 in]
    n167 = call-poly <vilib>:"Digital Write.vi"("Error In"=w285, "Values"="Values", "DO Channels"=u8[] [24, 49, 51, 53], "LINX Resource"=w286) -> ("Error Out"=w284:errorcluster, "LINX Resource"=w283:T7)  [unwired: 6 in]
    n168 = Or(x=w284, y="STOP") -> (x .or. y?=w295:bool)
  }
  n169 = while {
    tunnel: [w297] -> w8
    tunnel: "Servo Slider 1 Pin" -> [w297]
    tunnel: "Servo Slider 2 Pin" -> [w296]
    tunnel: [w296] -> w5
    tunnel: [w298] -> w4
    tunnel: "Servo Magazine Pin" -> [w298]
    shift-right: [w301] -> w10
    shift-left: w12 -> [w303]
    shift-right: [w300] -> w9
    shift-left: w11 -> [w302]
    stop <- w299 stop-if-true
    # "Servo Slider 2"
    # "Servo Slider 1"
    # "Servo Linear Actuator"
    # "Servo Control"
    n170 = Multiply(x="Servo Magazine Angle", y=u16 14) -> (x*y=w312:u16)
    n171 = call-poly <vilib>:"Servo Set Pulse Width.vi"("Error In"=w302, "Pulse Width (uS)"=w312, "Servo Channel"=w298, "LINX Resource"=w303) -> ("Error Out"=w308:errorcluster, "LINX Resource"=w307:T7)  [unwired: 6 in]
    n172 = Multiply(x="Servo Slider 1 Angle", y=u16 14) -> (x*y=w314:u16)
    n173 = call-poly <vilib>:"Servo Set Pulse Width.vi"("Error In"=w308, "Pulse Width (uS)"=w314, "Servo Channel"=w297, "LINX Resource"=w307) -> ("Error Out"=w310:errorcluster, "LINX Resource"=w309:T7)  [unwired: 6 in]
    n174 = Multiply(x="Servo Slider 2 Angle", y=u16 14) -> (x*y=w316:u16)
    n175 = call-poly <vilib>:"Servo Set Pulse Width.vi"("Error In"=w310, "Pulse Width (uS)"=w316, "Servo Channel"=w296, "LINX Resource"=w309) -> ("Error Out"=w300:errorcluster, "LINX Resource"=w301:T7)  [unwired: 6 in]
    n176 = local read "STOP"() -> (w299:bool)
  }
  n177 = Build Array(w8, w5, w4) -> (w14:u8[])
  n178 = call <vilib>:"Close.vi"("Error In"=w21, "LINX Resource"=w22) -> ()  [unwired: 9 in, 1 out]
  n179 = call-poly <vilib>:"Servo Close.vi"("Error In"=w9, "Servo Channels"=w14, "LINX Resource"=w10) -> ("Error Out"=w15:errorcluster, "LINX Resource"=w16:T7)  [unwired: 7 in]
  n180 = call <vilib>:"Close.vi"("Error In"=w15, "LINX Resource"=w16) -> ()  [unwired: 9 in, 1 out]
